vi "Shoot Spike (Auto).vi"(11 "Execute?":bool) -> (3 "Done":bool)   [LabVIEW 2012]
uses:
  <vilib>/Rock Robotics/WPI/Relay/WPI_RelayValue.ctl
  Globals/Log Data.vi
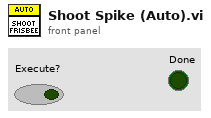
[diagram p1: front panel]
types:
  T1 = typedef "WPI_RelayDevRef.ctl" = cluster{"DevStatus":errorcluster, "Relay Channel":T2, "Digital Module":T3, "Relay Direction":T4}
  T2 = typedef "FPGA_DIORelayChannel.ctl" = enum8{"Relay 1", "Relay 2", "Relay 3", "Relay 4", "Relay 5", "Relay 6", "Relay 7", "Relay 8", "Invalid"}
  T3 = typedef "FPGA_TypedefDigitalModule.ctl" = enum16{"Digital Module 1", "Digital Module 2"}
  T4 = typedef "WPI_RelayDirection.ctl" = enum16{"Both directions", "Forward only", "Reverse only"}
  T5 = typedef "WPI_RelayValue.ctl" = enum16{"Off", "On", "Forward", "Reverse"}
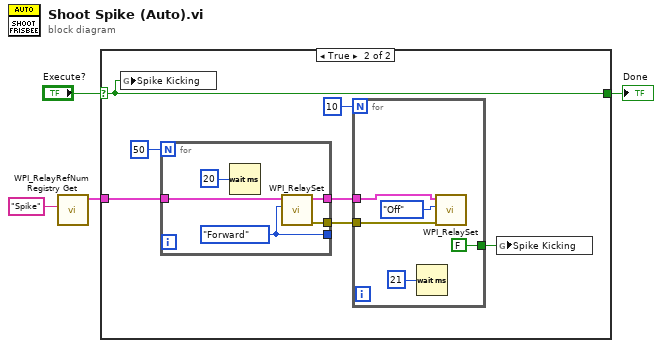
[diagram p0: block diagram]
diagram:
  n1 = call <vilib>:"WPI_RelayRefNum Registry Get.vi"("refnum name"="Spike") -> ("RelayDevRef"=w1:T1)  [unwired: 9 in, 1 out]
  n2 = case shown="True" "Execute?" {
    selector: "Execute?" -> [w5 w8]
    tunnel: [w5 w8] -> w3
    tunnel: w1 -> [_ w11]
    frame False {
    }
    frame True {
      n3 = global write "Log Data.vi" "Spike Kicking"(w8) -> ()
      n4 = for {
        N: 50 -> [_]
        tunnel: w11 -> [w21]
        tunnel: [w20] -> w10
        tunnel: [w19] -> _
        tunnel: [w18] -> w6
        w19 = WPI_RelayValue."Forward" ("RelayValue")
        n5 = Wait (ms)(milliseconds to wait=u32 20) -> ()  [unwired: 1 out]
        n6 = call <vilib>:"WPI_RelaySet.vi"("RelayValue"=w19, "RelayDevRef"=w21) -> ("error out"=w18:errorcluster, "RelayDevRef"=w20:T1)  [unwired: 8 in]
      }
      n7 = for {
        N: 10 -> [_]
        tunnel: w10 -> [w16]
        tunnel: [FALSE ("Spike Kicking")] -> w7
        tunnel: w6 -> [w13]
        n8 = Wait (ms)(milliseconds to wait=u32 21) -> ()  [unwired: 1 out]
        n9 = call <vilib>:"WPI_RelaySet.vi"("error in (no error)"=w13, "RelayValue"=WPI_RelayValue."Off", "RelayDevRef"=w16) -> ()  [unwired: 7 in, 2 out]
      }
      n10 = global write "Log Data.vi" "Spike Kicking"(w7) -> ()
    }
  }
  "Done" <- w3
